vi "cam2_cont.vi"() -> ()   [LabVIEW 2013]
uses:
  <vilib>/userdefined/High Color/IMAQdx.ctl
  <vilib>/vision/driver/NI_Vision_Acquisition_Software.lvlib
panel:
  in  "Camera":T1="cam0"
  out "Image":T2(plugin-control)
  out "Camera Information Array":T3(array[cluster]) {"BusType" format="%x"; "SerialNumberLow" format="%.0x"; "SerialNumberHigh" format="%.0x"}
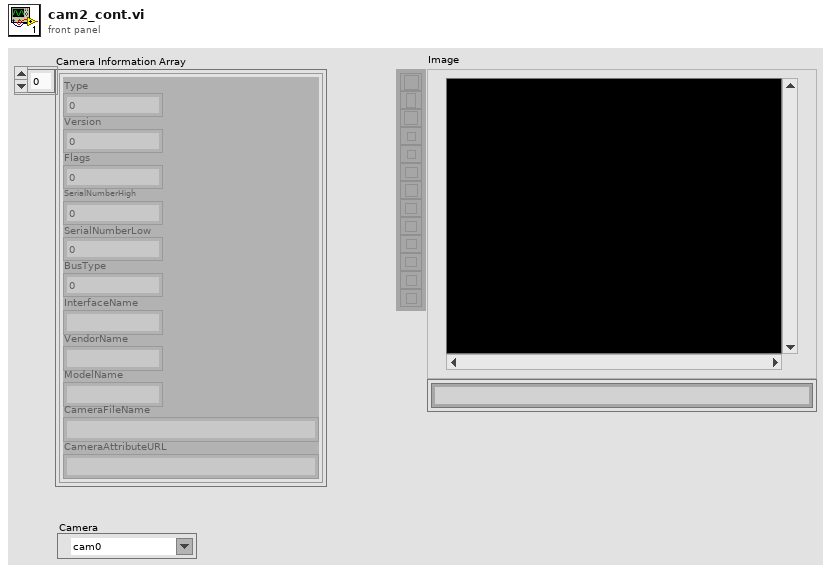
[diagram p1: front panel]
types:
  T1 = typedef "IMAQdx.ctl" = refnum<k21>
  T2 = typedef "IMAQ Image.ctl" = refnum<image>
  T3 = cluster{"Type":u32, "Version":u32, "Flags":u32, "SerialNumberHigh":u32, "SerialNumberLow":u32, "BusType":u32, "InterfaceName":string, "VendorName":string, "ModelName":string, "CameraFileName":string, "CameraAttributeURL":string}[]
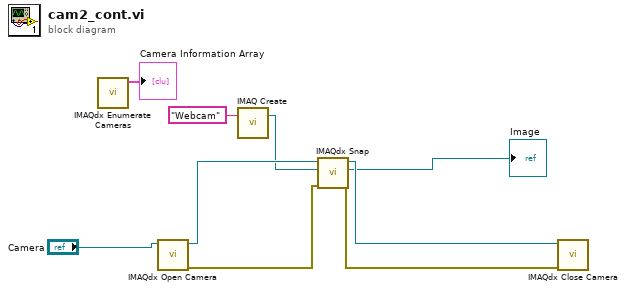
[diagram p0: block diagram]
diagram:
  n1 = call <vilib>:"IMAQdx Enumerate Cameras.vi"() -> ("Camera Information Array"=→"Camera Information Array":T3)  [unwired: 10 in, 1 out]
  n2 = call <vilib>:"IMAQdx Open Camera.vi"("Session In"="Camera") -> ("error out"=w6:errorcluster, "Session Out"=w8:T1)  [unwired: 9 in]
  n3 = call "IMAQ Create"("Image Name"="Webcam") -> ("New Image"=w3:T2)  [unwired: 4 in, 1 out]
  n4 = call <vilib>:"IMAQdx Snap.vi"("error in"=w6, "Image In"=w3, "Session In"=w8) -> ("error out"=w5:errorcluster, "Image Out"=→"Image":T2, "Session Out"=w7:T1)  [unwired: 6 in]
  n5 = call <vilib>:"IMAQdx Close Camera.vi"("error in"=w5, "Session In"=w7) -> ()  [unwired: 9 in, 1 out]
